vi "DAQ-AmpAdjustValue.vi"(1 "Limites":T1, 2 "Input":dbl) -> (0 "Output":dbl)   [LabVIEW 2010]
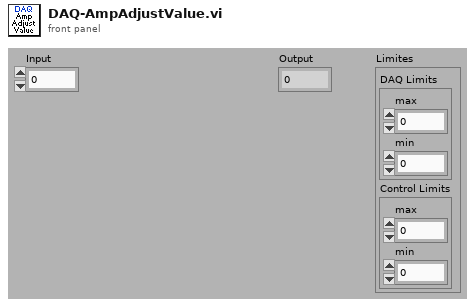
[diagram p1: front panel]
types:
  T1 = cluster{"DAQ Limits":cluster{"max":dbl, "min":dbl}, "Control Limits":cluster{"max":dbl, "min":dbl}}
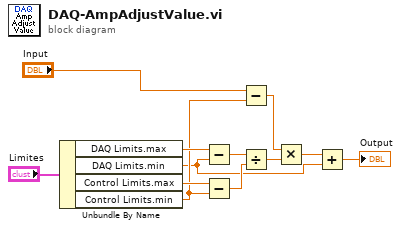
[diagram p0: block diagram]
diagram:
  n1 = Unbundle By Name("Limites") -> ("DAQ Limits.max"=w11:dbl, "DAQ Limits.min"=w4:dbl, "Control Limits.max"=w10:dbl, "Control Limits.min"=w9:dbl)
  n2 = Subtract(x=w11, y=w4) -> (x-y=w8:dbl)
  n3 = Subtract(x=w10, y=w9) -> (x-y=w7:dbl)
  n4 = Subtract(x="Input", y=w9) -> (x-y=w5:dbl)
  n5 = Divide(x=w8, y=w7) -> (x/y=w6:dbl)
  n6 = Multiply(x=w5, y=w6) -> (x*y=w3:dbl)
  n7 = Add(x=w3, y=w4) -> (x+y=→"Output":dbl)
